vi "Write WaitParams.vi"(8 "error in":errorcluster, 10 "WaitParams":cluster{"Timeout (ms)":u32, "LoopTime (ms)":u32}={"Timeout (ms)"=100, "LoopTime (ms)"=10}, 11 "Serial IO in":refnum<class "Serial IO.lvclass">) -> (0 "error out":errorcluster, 3 "Serial IO out":refnum<class "Serial IO.lvclass">)   [LabVIEW 2015, in "Serial IO.lvclass"]
doc: "Write the parameters use to poll the serial device. <B>Timeout (ms)</B> will set the total amount of time to poll the device (default is 100 ms) while <B>LoopTime (ms)</B> sets the rate at which the device is polled (10 ms is the default)."
uses:
  Serial IO.lvclass
  Serial IO.lvclass/Serial IO.ctl
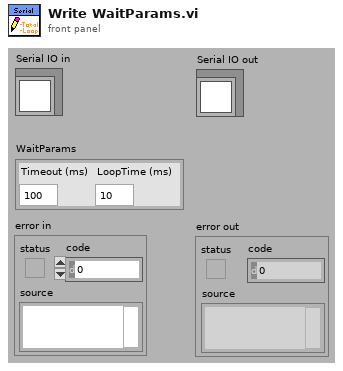
[diagram p1: front panel]
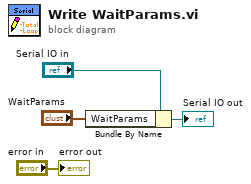
[diagram p0: block diagram]
diagram:
  n1 = Bundle By Name(cluster="Serial IO in", "WaitParams"="WaitParams") -> (→"Serial IO out":refnum<class "Serial IO.lvclass">)
  "error out" <- "error in"
